vi "fgv_nonlinearRamps.vi"(8 "error in (no error)":errorcluster, 10 "Status":enum16{"Initialize", "Write", "Read"}(ring), 11 "C,D,E Parameters In":T1) -> (0 "error out":errorcluster, 1 "C,D,E Array":dbl[](array[numeric]), 3 "C,D,E Parameters Out":T1)   [LabVIEW 2017]
uses:
  Acquisition/Typedefs/nonlinearRamps_CDE.ctl
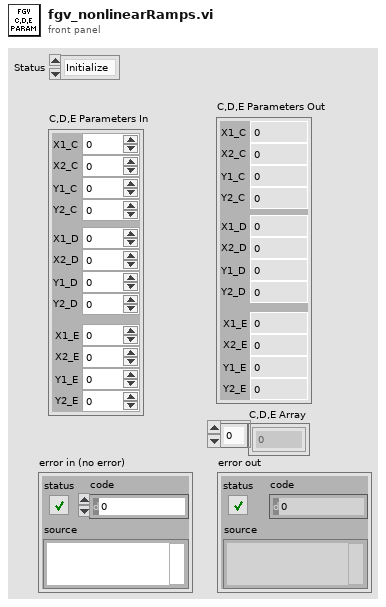
[diagram p1: front panel]
types:
  T1 = typedef "nonlinearRamps_CDE.ctl" = cluster{"X1_C":dbl, "X2_C":dbl, "Y1_C":dbl, "Y2_C":dbl, "X1_D":dbl, "X2_D":dbl, "Y1_D":dbl, "Y2_D":dbl, "X1_E":dbl, "X2_E":dbl, "Y1_E":dbl, "Y2_E":dbl}
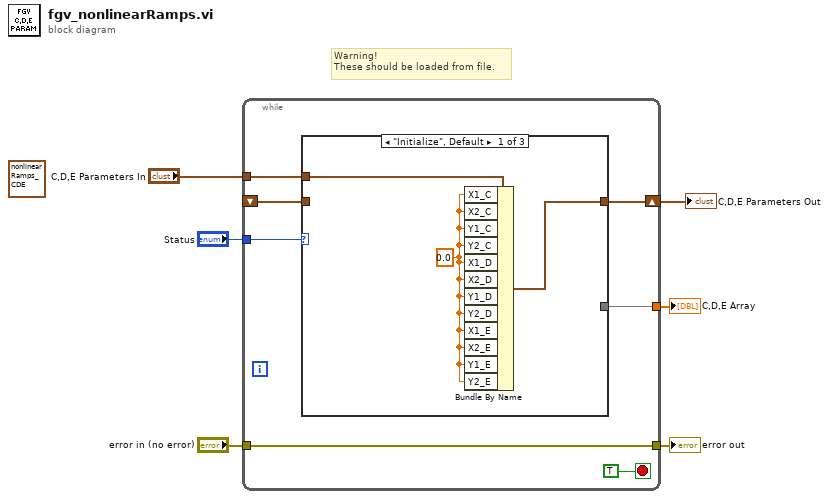
[diagram p0: block diagram]
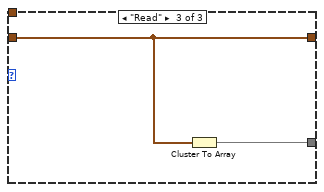
[diagram p3: hidden frame]
diagram:
  (unwired) T1 {"X1_C"=0.0, "X2_C"=0.0, "Y1_C"=0.0, "Y2_C"=0.0, "X1_D"=0.0, "X2_D"=0.0, "Y1_D"=0.0, "Y2_D"=0.0, "X1_E"=0.0, "X2_E"=0.0, "Y1_E"=0.0, "Y2_E"=0.0} ("C,D,E Parameters In")
  # "Warning!\nThese should be loaded from file."
  n1 = while {
    tunnel: "Status" -> [w12]
    shift-right: [w11] -> w2
    shift-left: _ -> [w10]
    tunnel: "C,D,E Parameters In" -> [w9]
    tunnel: "error in (no error)" -> [w8]
    tunnel: [w8] -> w4
    tunnel: [w7] -> w1
    stop <- TRUE stop-if-true
    n2 = case shown="\"Initialize\", Default" w12 {
      tunnel: [w15 w17 w19] -> w11
      tunnel: w10 -> [_ _ w19]
      tunnel: w9 -> [w16 w17 _]
      tunnel: [_ _ w18] -> w7
      frame "Initialize", Default {
        w14 = 0.0 ("Ref_dwellTime")
        n3 = Bundle By Name(cluster=w16, "X1_C"=w14, "X2_C"=w14, "Y1_C"=w14, "Y2_C"=w14, "X1_D"=w14, "X2_D"=w14, "Y1_D"=w14, "Y2_D"=w14, "X1_E"=w14, "X2_E"=w14, "Y1_E"=w14, "Y2_E"=w14) -> (w15:T1)
      }
      frame "Write" {
      }
      frame "Read" {
        n4 = Cluster To Array(cluster=w19) -> (array=w18:dbl[])
      }
    }
  }
  "error out" <- w4
  "C,D,E Parameters Out" <- w2
  "C,D,E Array" <- w1
